vi "IMAQdx_GetCameraInformation.vi"(8 "error in (no error)":errorcluster caption="错误输入（无错误）", 11 "Connected Only? (Yes)":bool) -> (0 "error out":errorcluster caption="错误输出", 2 "Camera Basic Information":string[][](array[string]), 3 "Camera Information Array":T1(array[cluster]) {"BusType" format="%x"; "SerialNumberLow" format="%.0x"; "SerialNumberHigh" format="%.0x"})   [LabVIEW 2015]
uses:
  <vilib>/vision/driver/NI_Vision_Acquisition_Software.lvlib
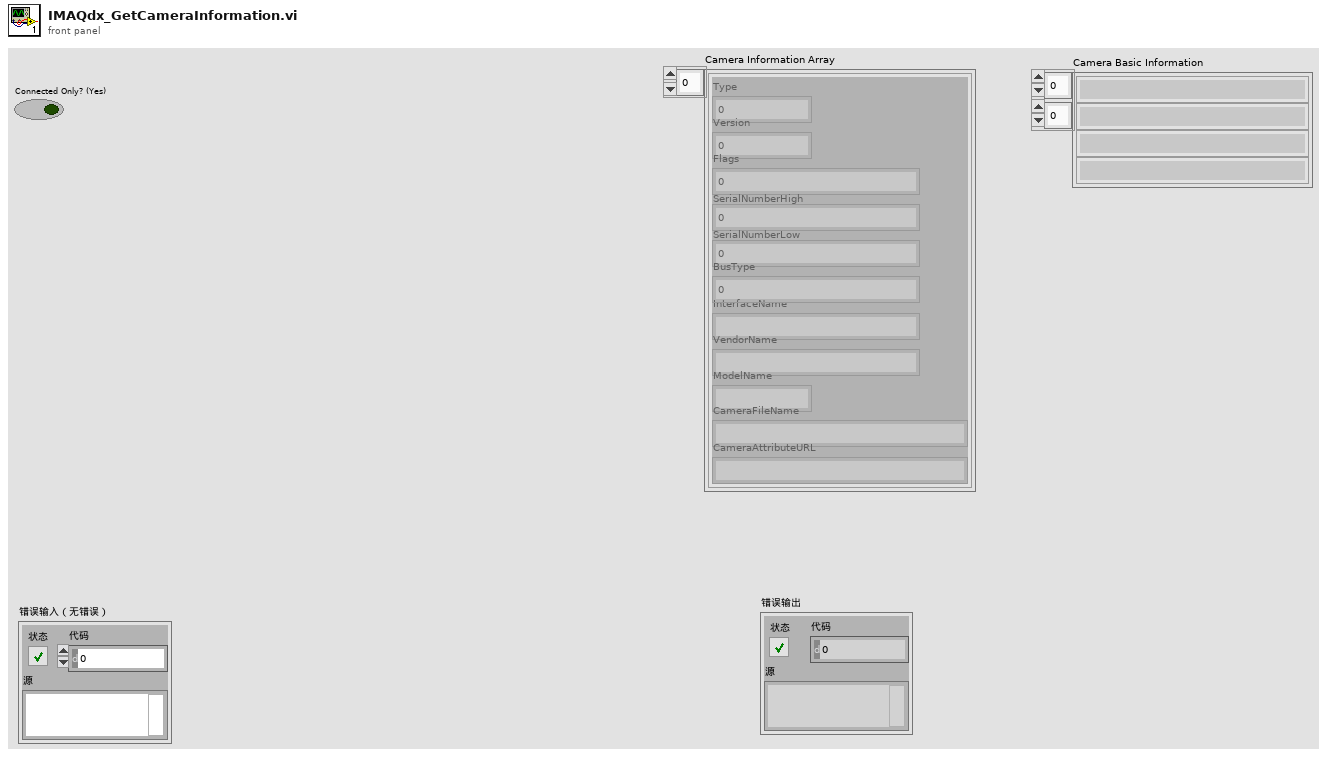
[diagram p1: front panel]
types:
  T1 = cluster{"Type":u32, "Version":u32, "Flags":u32, "SerialNumberHigh":u32, "SerialNumberLow":u32, "BusType":u32, "InterfaceName":string, "VendorName":string, "ModelName":string, "CameraFileName":string, "CameraAttributeURL":string}[]
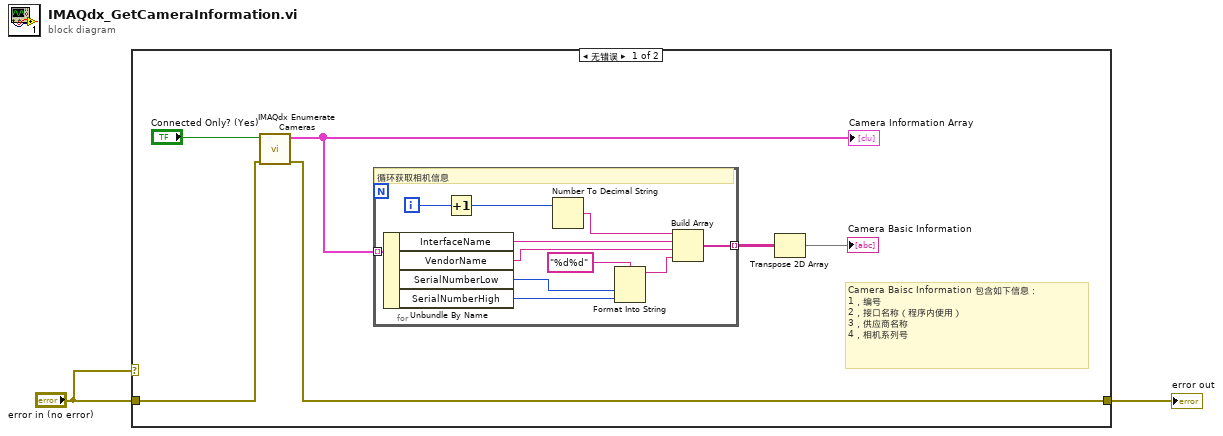
[diagram p0: block diagram]
diagram:
  n1 = case shown="无错误" "error in (no error)" {
    tunnel: "error in (no error)" -> [w4 w20]
    tunnel: [w3 w20] -> w2
    frame No Error {
      # "Camera Baisc Information 包含如下信息：\n1，编号\n2，接口名称（程序内使用）\n3，供应商名称\n4，相机系列号"
      n2 = call <vilib>:"IMAQdx Enumerate Cameras.vi"("error in"=w4, "Connected Only? (Yes)"="Connected Only? (Yes)") -> ("error out"=w3:errorcluster, "Camera Information Array"=w7:T1)  [unwired: 8 in]
      "Camera Information Array" <- w7
      n3 = for {
        tunnel: w7 -> [w19] mode=indexing
        tunnel: [w13] -> w6 mode=indexing
        i -> [w18]
        # "循环获取相机信息"
        n4 = Unbundle By Name(w19) -> ("InterfaceName"=w15:string, "VendorName"=w14:string, "SerialNumberLow"=w12:u32, "SerialNumberHigh"=w11:u32)
        n5 = Increment(x=w18) -> (x+1=w16:i32)
        n6 = Number To Decimal String(number=w16) -> (decimal integer string=w17:string)  [unwired: 1 in]
        n7 = Format Into String(format string="%d%d" ("初始字符串"), w12, w11) -> (resulting string=w10:string)  [unwired: 2 in, 1 out]
        n8 = Build Array(w17, w15, w14, w10) -> (w13:string[])
      }
      n9 = Transpose 2D Array(2D array=w6) -> (transposed array=→"Camera Basic Information":string[][])
    }
    frame Error {
    }
  }
  "error out" <- w2
